vi "PruebaSequence.vi"() -> ()   [LabVIEW 2014, in "MSX-E3711.lvlib"]
uses:
  MSX-E3711Class/MSX-E3711.lvlib
  MSX-E3711Class/MSX-E3711.lvclass
panel:
  out "Array":sgl[](array[numeric]) format="%#_6f"
  in  "stop":bool
  out "TODO":sgl[][](array[numeric]) format="%#.5f"
  out "Muestras por seg":dbl
  out "Segundos":dbl
  out "Muestras":i32
  out "error out":errorcluster
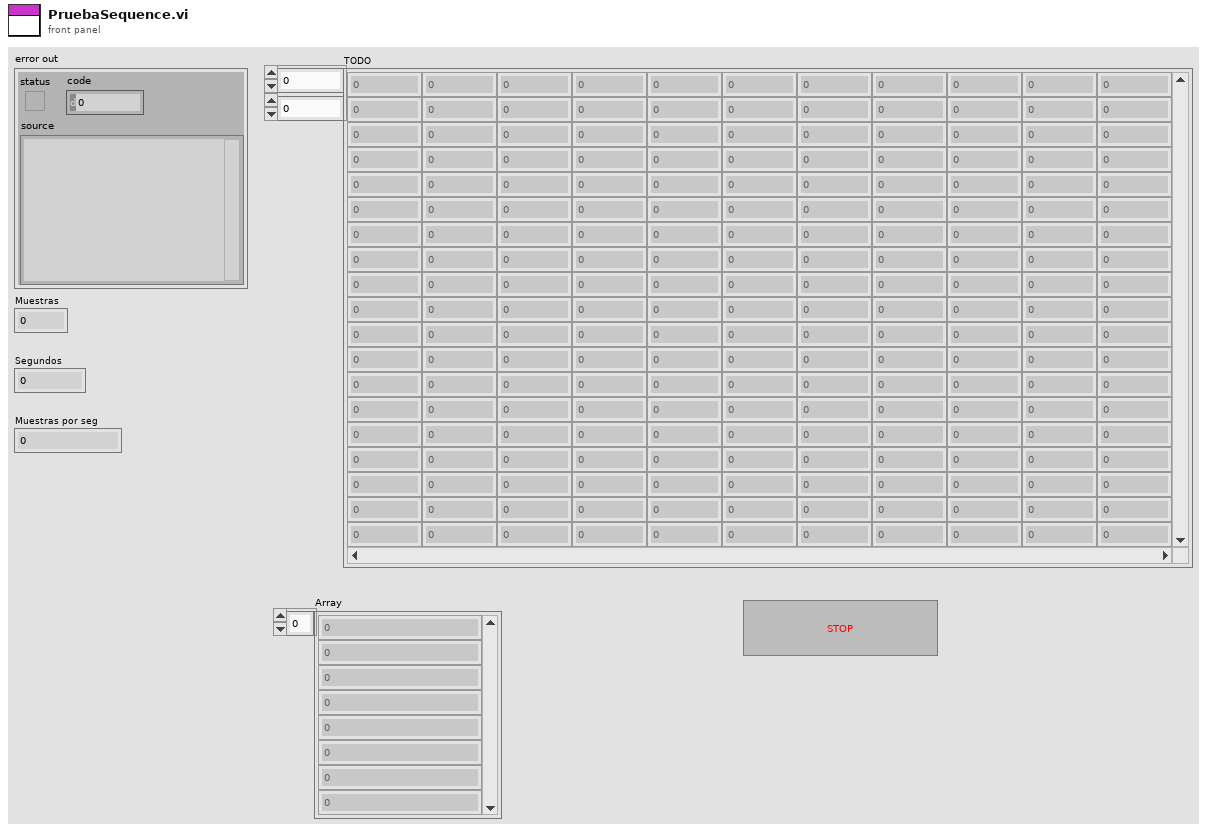
[diagram p1: front panel]
types:
  T1 = typedef "DriverMasterSync.lvlibp/WINFAS 2 Data Queue.lvlib/Acquisition Data 1 Sample Cluster.ctl" = cluster{"TDX":sgl[], "Encoder":sgl}
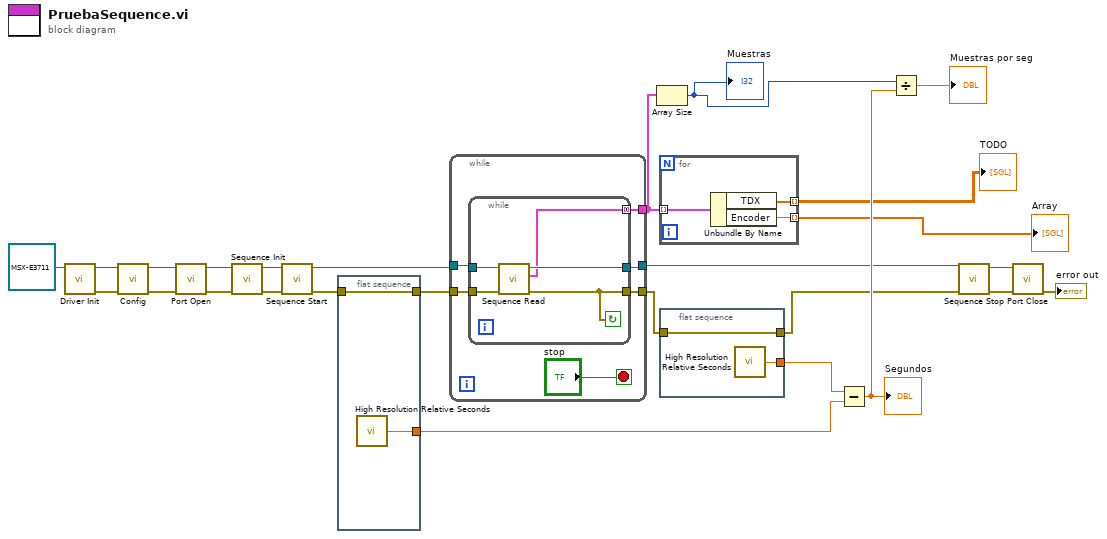
[diagram p0: block diagram]
diagram:
  n1 = call-dynamic "Driver Init.vi"("MSX-E3711 in"=refnum<class "MSX-E3711.lvclass"> refnum) -> ("error out"=w16:errorcluster, "MSX-E3711 out"=w26:refnum<class "MSX-E3711.lvclass">)  [unwired: 9 in]
  n2 = call-dynamic "Config.vi"("error in (no error)"=w16, "MSX-E3711 in"=w26) -> ("error out"=w17:errorcluster, "MSX-E3711 out"=w25:refnum<class "MSX-E3711.lvclass">)  [unwired: 7 in, 1 out]
  n3 = call-dynamic "Port Open.vi"("error in (no error)"=w17, "MSX-E3711 in"=w25) -> ("error out"=w18:errorcluster, "MSX-E3711 out"=w24:refnum<class "MSX-E3711.lvclass">)  [unwired: 8 in]
  n4 = call-dynamic "Sequence Init.vi"("error in (no error)"=w18, "MSX-E3711 in"=w24) -> ("error out"=w19:errorcluster, "MSX-E3711 out"=w23:refnum<class "MSX-E3711.lvclass">)  [unwired: 8 in]
  n5 = call-dynamic "Sequence Start.vi"("error in (no error)"=w19, "MSX-E3711 in"=w23) -> ("error out"=w8:errorcluster, "MSX-E3711 out"=w22:refnum<class "MSX-E3711.lvclass">)  [unwired: 8 in]
  n6 = flat-sequence {
    tunnel: [w28] -> w7
    tunnel: w8 -> [w28]
    tunnel: [w27] -> w12
    frame #0 {
      n7 = call <vilib>:"High Resolution Relative Seconds.vi"() -> ("relative seconds"=w27:dbl)
    }
  }
  n8 = while {
    tunnel: [w30] -> w3
    tunnel: w22 -> [w34]
    tunnel: [w32] -> w6
    tunnel: w7 -> [w33]
    tunnel: [w31] -> w5
    stop <- "stop" stop-if-true
    n9 = while {
      tunnel: w34 -> [w39]
      tunnel: [w38] -> w32
      tunnel: [w36] -> w31
      tunnel: w33 -> [w37]
      tunnel: [w35] -> w30 mode=concatenating
      stop <- w36 continue-if-true
      n10 = call-dynamic "Sequence Read.vi"("error in (no error)"=w37, "MSX-E3711 in"=w39) -> ("error out"=w36:errorcluster, "Acquisition Data"=w35:T1[], "MSX-E3711 out"=w38:refnum<class "MSX-E3711.lvclass">)  [unwired: 6 in, 1 out]
    }
  }
  n11 = Array Size(array=w3) -> (size(s)=w9:i32)
  "Muestras" <- w9
  n12 = for {
    tunnel: w3 -> [w42] mode=indexing
    tunnel: [w41] -> w2 mode=indexing
    tunnel: [w40] -> w1 mode=indexing
    n13 = Unbundle By Name(w42) -> ("TDX"=w41:sgl[], "Encoder"=w40:sgl)
  }
  "TODO" <- w2
  "Array" <- w1
  n14 = flat-sequence {
    tunnel: [w44] -> w4
    tunnel: w5 -> [w44]
    tunnel: [w43] -> w13
    frame #0 {
      n15 = call <vilib>:"High Resolution Relative Seconds.vi"() -> ("relative seconds"=w43:dbl)
    }
  }
  n16 = Subtract(x=w13, y=w12) -> (x-y=w11:dbl)
  "Segundos" <- w11
  n17 = Divide(x=w9, y=w11) -> (x/y=→"Muestras por seg":dbl)
  n18 = call-dynamic "Sequence Stop.vi"("error in (no error)"=w4, "MSX-E3711 in"=w6) -> ("error out"=w20:errorcluster, "MSX-E3711 out"=w21:refnum<class "MSX-E3711.lvclass">)  [unwired: 8 in]
  n19 = call-dynamic "Port Close.vi"("error in (no error)"=w20, "MSX-E3711 in"=w21) -> ("error out"=→"error out":errorcluster)  [unwired: 8 in, 1 out]
